vi "Color Opacity Calc.vi"(9 "opacity":dbl, 10 "Original Color":u32(colorbox)) -> (2 "Modified Color":u32(colorbox))   [LabVIEW 2021, in "TSC Material Theme.lvlib" / "Material-Scheme.lvclass"]
doc: "apply an opacity percentage to a color\n\n<b>Note</b>: opacity input expected to be decimal of the percentage\n\n<b>Code Developed By:</b>\nTechnology Service Corporation\nwww.tsc.com/atcs\n\nDeveloper:\nDaniel Coons"
uses:
  Material-Scheme.lvclass
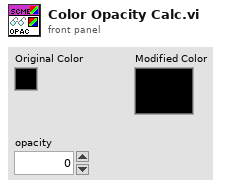
[diagram p1: front panel]
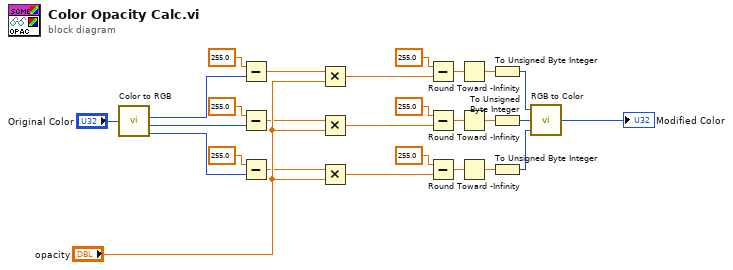
[diagram p0: block diagram]
diagram:
  n1 = call <vilib>:"Color to RGB.vi"("Color"="Original Color") -> ("R"=w2:u8, "G"=w22:u8, "B"=w23:u8)  [unwired: 1 out]
  n2 = Subtract(x=255.0, y=w2) -> (x-y=w3:dbl)
  n3 = Subtract(x=255.0, y=w22) -> (x-y=w14:dbl)
  n4 = Subtract(x=255.0, y=w23) -> (x-y=w17:dbl)
  n5 = Multiply(x=w3, y="opacity") -> (x*y=w5:dbl)
  n6 = Multiply(x=w14, y="opacity") -> (x*y=w12:dbl)
  n7 = Multiply(x=w17, y="opacity") -> (x*y=w19:dbl)
  n8 = Subtract(x=255.0, y=w5) -> (x-y=w6:dbl)
  n9 = Subtract(x=255.0, y=w12) -> (x-y=w11:dbl)
  n10 = Subtract(x=255.0, y=w19) -> (x-y=w20:dbl)
  n11 = Round Toward -Infinity(1:w6) -> (0:w7:dbl)
  n12 = Round Toward -Infinity(1:w11) -> (0:w10:dbl)
  n13 = Round Toward -Infinity(1:w20) -> (0:w21:dbl)
  n14 = To Unsigned Byte Integer(number=w7) -> (unsigned 8bit integer=w8:u8)
  n15 = To Unsigned Byte Integer(number=w10) -> (unsigned 8bit integer=w24:u8)
  n16 = To Unsigned Byte Integer(number=w21) -> (unsigned 8bit integer=w25:u8)
  n17 = call <vilib>:"RGB to Color.vi"("B"=w25, "G"=w24, "R"=w8) -> ("Color"=→"Modified Color":u32)
